vi "getTemperature.vi"(8 "error in (no error)":errorcluster, 11 "Camera in":refnum<class "Camera.lvclass">) -> (0 "error out":errorcluster, 2 "temperature":dbl, 3 "Camera out":refnum<class "Camera.lvclass">)   [LabVIEW 2011, in "Hardware.lvlib" / "Channels.lvlib" / "Camera.lvclass"]
uses:
  Camera.lvclass
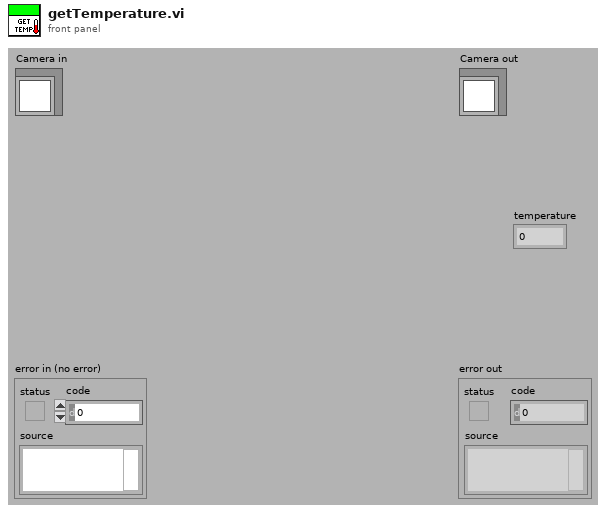
[diagram p1: front panel]
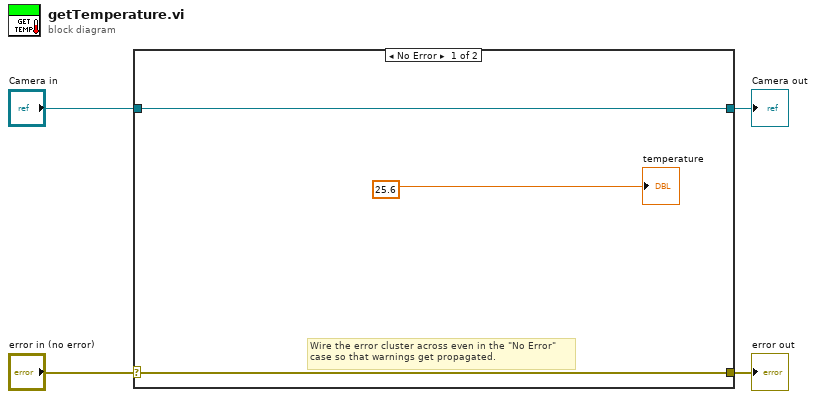
[diagram p0: block diagram]
diagram:
  n1 = case shown="No Error" "error in (no error)" {
    selector: "error in (no error)" -> [w6 w9]
    tunnel: [w6 w9] -> w3
    tunnel: [w7 w8] -> w1
    tunnel: "Camera in" -> [w7 w8]
    frame No Error {
      # "Wire the error cluster across even in the \"No Error\"\ncase so that warnings get propagated."
      "temperature" <- 25.6
    }
    frame Error {
    }
  }
  "error out" <- w3
  "Camera out" <- w1
